vi "file_name_generator.vi"() -> (3 "file_name":path)   [LabVIEW 2021]
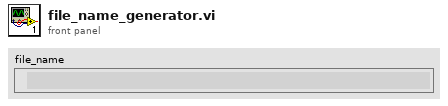
[diagram p1: front panel]
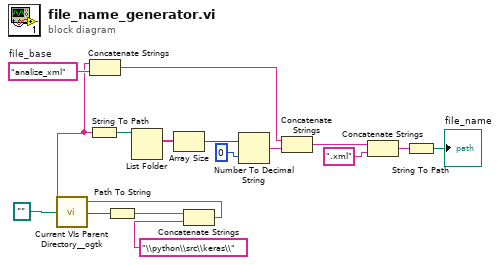
[diagram p0: block diagram]
diagram:
  w12 = "analize_xml"  # file_base
  n1 = call <userlib>:"Current VIs Parent Directory__ogtk.vi"("Relative path (.)"=path "") -> ("Parent Directory (+ Relative)"=w4:path)  [unwired: 4 in]
  n2 = Path To String(path=w4) -> (string=w3:string)
  n3 = Concatenate Strings(w3, "\\python\\src\\keras\\") -> (w1:string)
  n4 = String To Path(string=w1) -> (path=w16:path)
  n5 = Concatenate Strings(w1, w12) -> (w11:string)
  n6 = List Folder(path=w16) -> (filenames=w15:string[])  [unwired: 3 in, 3 out]
  n7 = Array Size(array=w15) -> (size(s)=w14:i32)
  n8 = Number To Decimal String(number=w14, width (-)=i16 0) -> (decimal integer string=w10:string)
  n9 = Concatenate Strings(w11, w10) -> (w7:string)
  n10 = Concatenate Strings(w7, ".xml" ("string")) -> (w8:string)
  n11 = String To Path(string=w8) -> (path=→"file_name":path)
